vi "pulse destrbute_tester_1.vi"() -> ()   [LabVIEW 2021]
uses:
  Program Files/National Instruments/LabVIEW 2022/instr.lib/_niInstr/DSP/v1/Shared/Public/IQ Data.ctl
  Program Files/National Instruments/LabVIEW 2022/instr.lib/_niInstr/DSP/v1/Shared/niInstr DSP v1 Shared.lvlib
  pdw.ctl
panel:
  out "result 3":bool
  out "result 2":bool
  out "result":bool
  out "DDS free":bool[](array[boolean])=[FALSE, FALSE, FALSE, FALSE, FALSE, FALSE, FALSE, FALSE, FALSE, FALSE, FALSE, FALSE, FALSE, FALSE, FALSE, TRUE]
  in  "PDW":T1={"PW"=20, "frequency shift"=0.0, "amp"=0.9999923706054688, "mode type"=0, "mode file"=0, "mode depth"=0, "filter rate_pulse"=0, "filter rate bpsk"=0} {"frequency shift" format="%#_12f"}
  out "loop #":i32=421
  in  "stop":bool
  in  "new poulse":bool=TRUE
  in  "time good":bool=TRUE
  out "get new poulse":bool=TRUE
  out "output cluster":T2
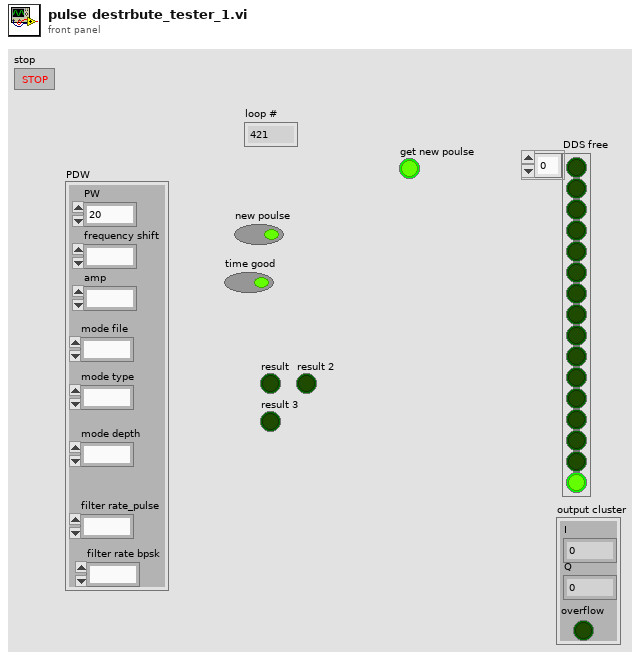
[diagram p1: front panel]
types:
  T1 = typedef "pdw.ctl" = cluster{"PW":u32, "frequency shift":fxp<+/-,48,0>, "amp":fxp<+/-,18,1>, "mode type":u8, "mode file":u8, "mode depth":u32, "filter rate_pulse":u16, "filter rate bpsk":u16}
  T2 = typedef "niInstr DSP v1 Shared.lvlib/IQ Data.ctl" = cluster{"I":fxp<+/-,18,1>, "Q":fxp<+/-,18,1>, "overflow":bool}
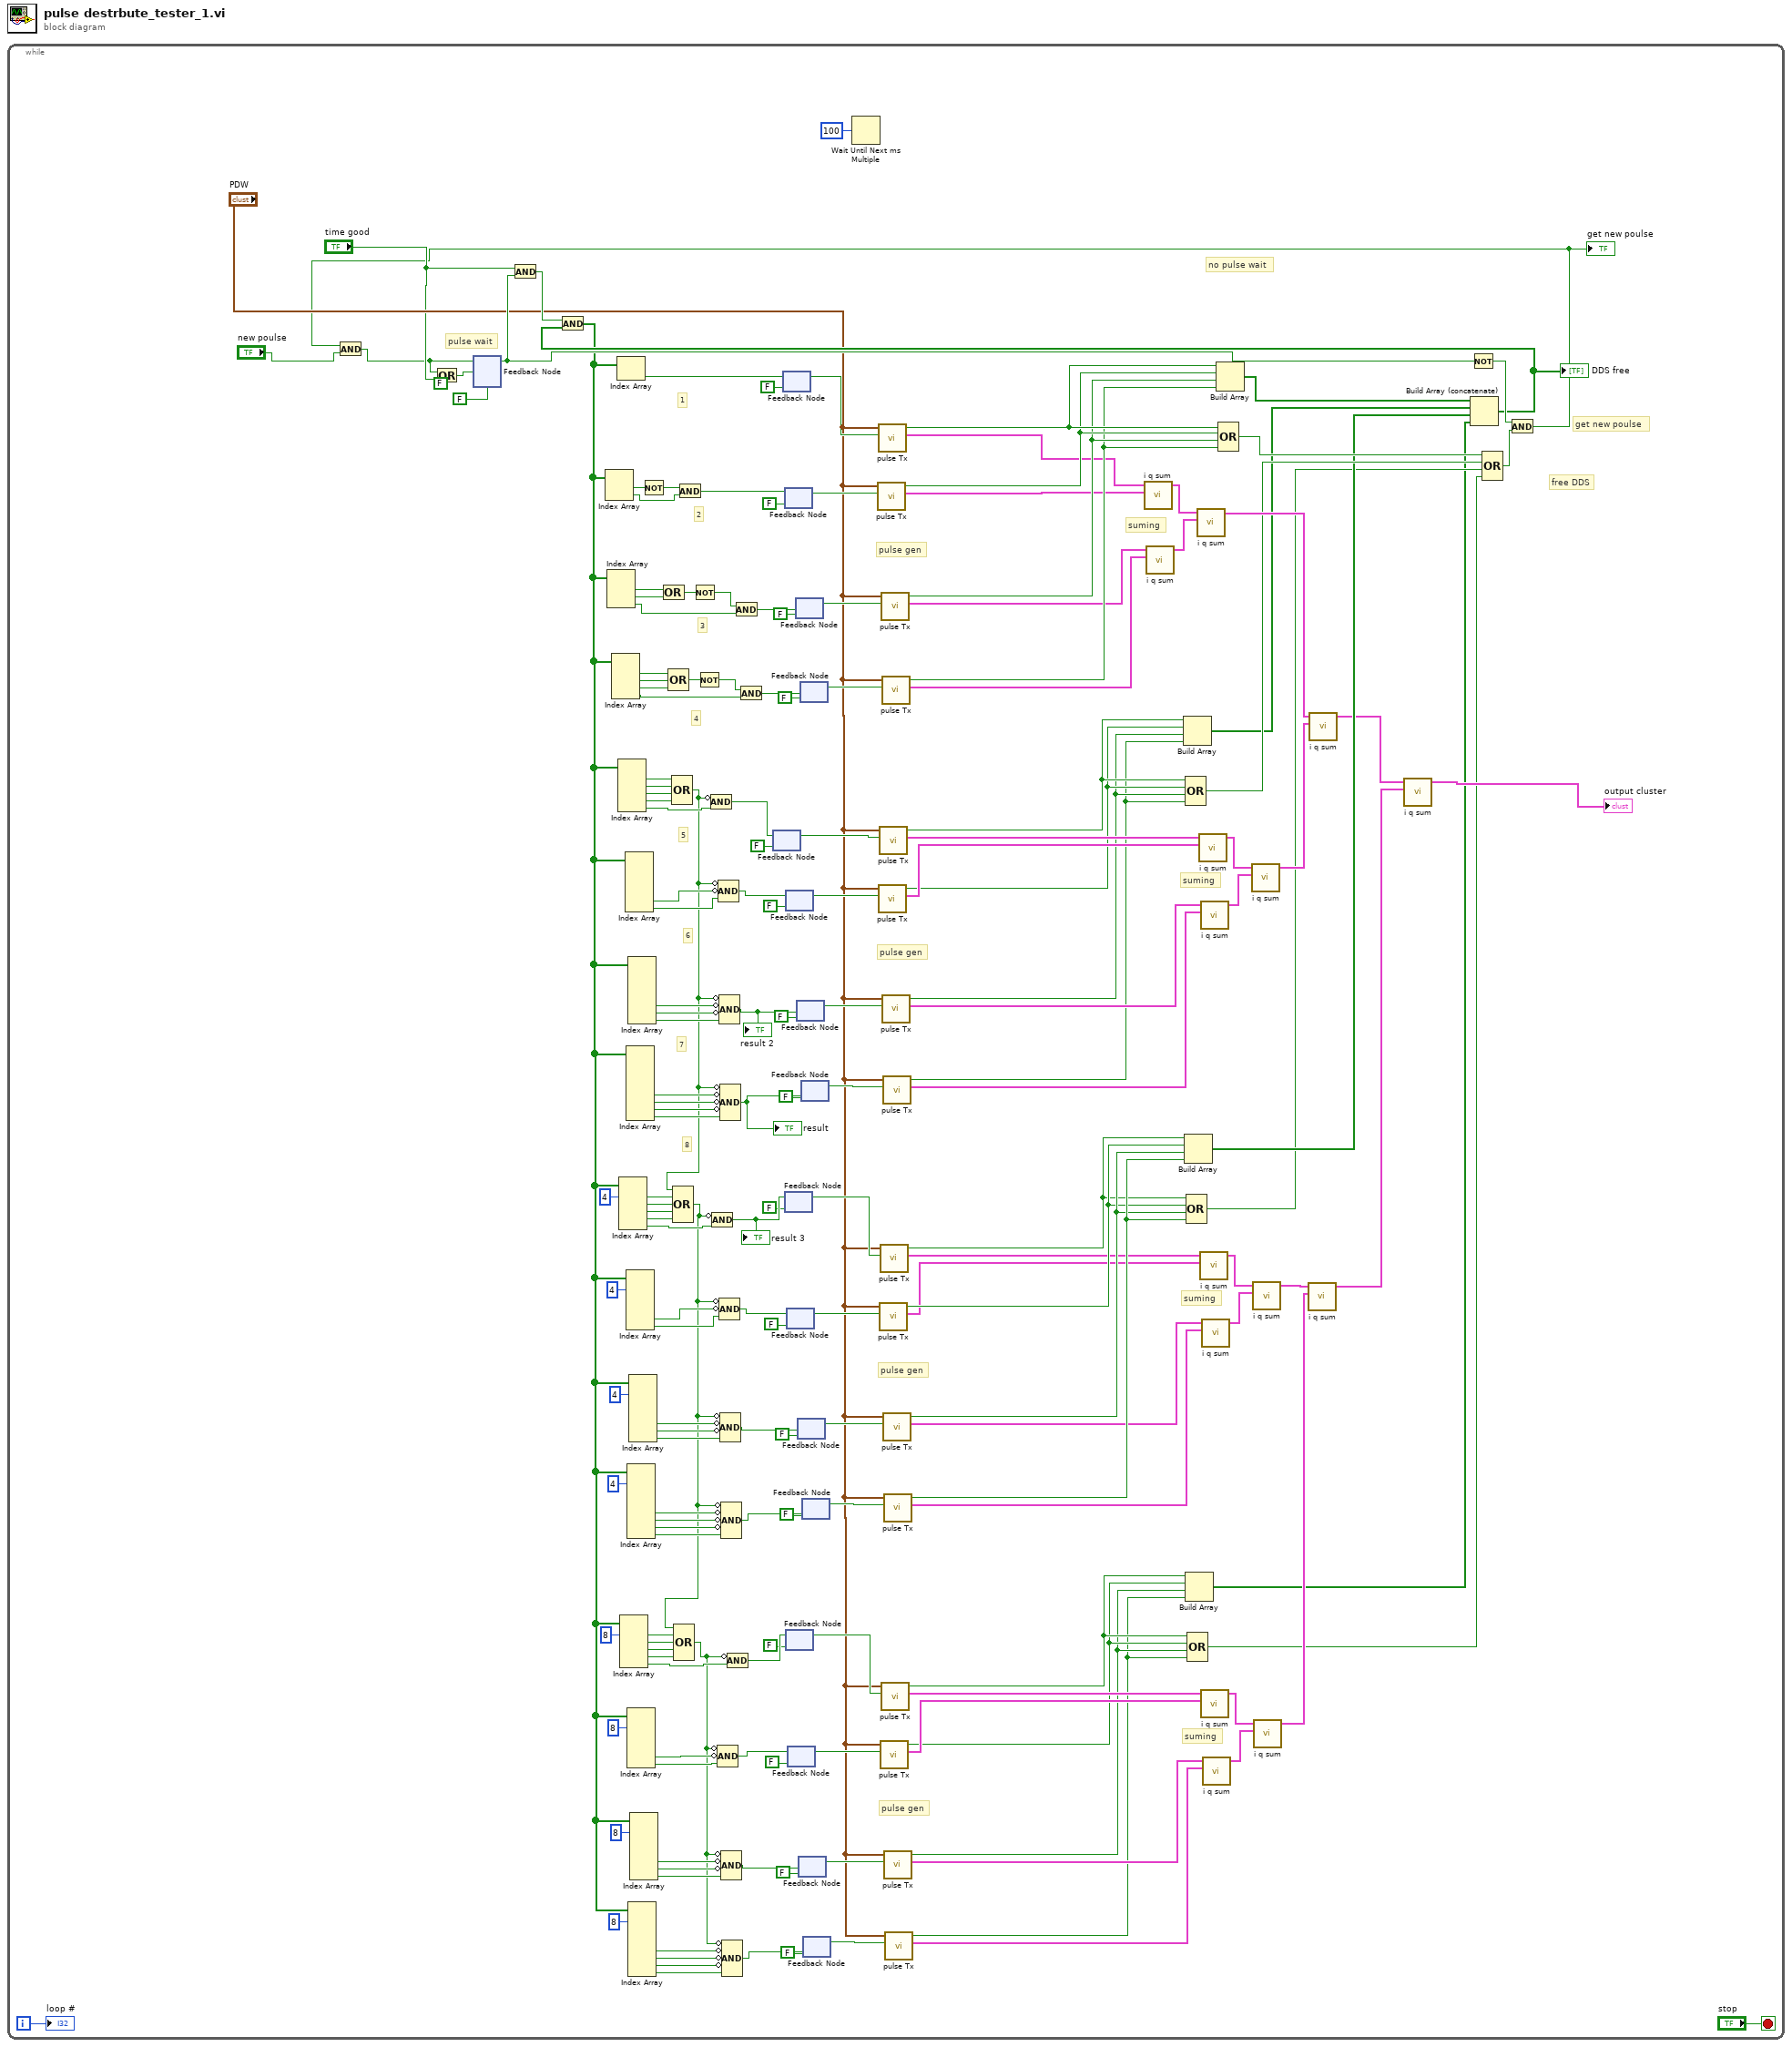
[diagram p0: block diagram]
diagram:
  n1 = while {
    i -> [w4]
    stop <- "stop" stop-if-true
    (unwired) FALSE ("Output Valid")
    # "8"
    # "7"
    # "6"
    # "5"
    # "4"
    # "3"
    # "2"
    # "1"
    # "suming"
    # "pulse gen"
    # "suming"
    # "pulse gen"
    # "suming"
    # "pulse gen"
    # "pulse wait"
    # "suming"
    # "pulse gen"
    # "get new poulse"
    # "no pulse wait"
    # "free DDS"
    n2 = feedback #1(FALSE ("Output Valid")) -> (w150:bool)
    n3 = And(x="time good", y=w150) -> (x .and. y?=w161:bool)
    n4 = feedback #2(FALSE) -> (w149:bool)
    n5 = feedback #3(FALSE) -> (w153:bool)
    n6 = feedback #4(FALSE) -> (w173:bool)
    n7 = feedback #5(FALSE) -> (w78:bool)
    n8 = feedback #6(FALSE) -> (w146:bool)
    n9 = feedback #7(FALSE) -> (w64:bool)
    n10 = feedback #8(FALSE) -> (w81:bool)
    n11 = feedback #9(FALSE) -> (w61:bool)
    n12 = feedback #10(FALSE) -> (w172:bool)
    n13 = feedback #11(FALSE) -> (w147:bool)
    n14 = feedback #12(FALSE) -> (w80:bool)
    n15 = feedback #13(FALSE) -> (w62:bool)
    n16 = feedback #14(FALSE) -> (w170:bool)
    n17 = feedback #15(FALSE) -> (w148:bool)
    n18 = feedback #16(FALSE) -> (w79:bool)
    n19 = feedback #17(FALSE) -> (w63:bool)
    n20 = Wait Until Next ms Multiple(millisecond multiple=u32 100) -> ()  [unwired: 1 out]
    n21 = call "pulse Tx.vi"("take it!"=w173, "Cluster"="PDW") -> ("data out"=w158:T2, "free dds"=w185:bool)  [unwired: 5 in, 3 out]
    n22 = call "pulse Tx.vi"("take it!"=w153, "Cluster"="PDW") -> ("data out"=w159:T2, "free dds"=w186:bool)  [unwired: 5 in, 3 out]
    n23 = call "pulse Tx.vi"("take it!"=w146, "Cluster"="PDW") -> ("data out"=w142:T2, "free dds"=w118:bool)  [unwired: 5 in, 3 out]
    n24 = call "pulse Tx.vi"("take it!"=w149, "Cluster"="PDW") -> ("data out"=w143:T2, "free dds"=w119:bool)  [unwired: 5 in, 3 out]
    n25 = call "pulse Tx.vi"("take it!"=w81, "Cluster"="PDW") -> ("data out"=w85:T2, "free dds"=w107:bool)  [unwired: 5 in, 3 out]
    n26 = call "pulse Tx.vi"("take it!"=w78, "Cluster"="PDW") -> ("data out"=w84:T2, "free dds"=w106:bool)  [unwired: 5 in, 3 out]
    n27 = call "pulse Tx.vi"("take it!"=w61, "Cluster"="PDW") -> ("data out"=w57:T2, "free dds"=w34:bool)  [unwired: 5 in, 3 out]
    n28 = call "pulse Tx.vi"("take it!"=w172, "Cluster"="PDW") -> ("data out"=w157:T2, "free dds"=w171:bool)  [unwired: 5 in, 3 out]
    n29 = call "pulse Tx.vi"("take it!"=w64, "Cluster"="PDW") -> ("data out"=w58:T2, "free dds"=w35:bool)  [unwired: 5 in, 3 out]
    n30 = call "pulse Tx.vi"("take it!"=w170, "Cluster"="PDW") -> ("data out"=w156:T2, "free dds"=w162:bool)  [unwired: 5 in, 3 out]
    n31 = call "pulse Tx.vi"("take it!"=w147, "Cluster"="PDW") -> ("data out"=w141:T2, "free dds"=w117:bool)  [unwired: 5 in, 3 out]
    n32 = call "pulse Tx.vi"("take it!"=w148, "Cluster"="PDW") -> ("data out"=w140:T2, "free dds"=w116:bool)  [unwired: 5 in, 3 out]
    n33 = call "pulse Tx.vi"("take it!"=w80, "Cluster"="PDW") -> ("data out"=w86:T2, "free dds"=w108:bool)  [unwired: 5 in, 3 out]
    n34 = call "pulse Tx.vi"("take it!"=w79, "Cluster"="PDW") -> ("data out"=w87:T2, "free dds"=w109:bool)  [unwired: 5 in, 3 out]
    n35 = call "pulse Tx.vi"("take it!"=w62, "Cluster"="PDW") -> ("data out"=w56:T2, "free dds"=w33:bool)  [unwired: 5 in, 3 out]
    n36 = call "pulse Tx.vi"("take it!"=w63, "Cluster"="PDW") -> ("data out"=w55:T2, "free dds"=w32:bool)  [unwired: 5 in, 3 out]
    n37 = call "i q sum.vi"(10:"data in"=w158, 11:"data in"=w159) -> ("output cluster"=w155:T2)  [unwired: 8 in, 1 out]
    n38 = call "i q sum.vi"(10:"data in"=w156, 11:"data in"=w157) -> ("output cluster"=w154:T2)  [unwired: 8 in, 1 out]
    n39 = Build Array(w119, w118, w117, w116) -> (w111:bool[])
    n40 = Build Array(w106, w107, w108, w109) -> (w72:bool[])
    n41 = Compound Arithmetic op=OR(w119, w118, w117, w116) -> (w114:bool)
    n42 = Build Array(w35, w34, w33, w32) -> (w27:bool[])
    n43 = Compound Arithmetic op=OR(w106, w107, w108, w109) -> (w71:bool)
    n44 = Compound Arithmetic op=OR(w35, w34, w33, w32) -> (w26:bool)
    n45 = call "i q sum.vi"(10:"data in"=w154, 11:"data in"=w155) -> ("output cluster"=w121:T2)  [unwired: 8 in, 1 out]
    n46 = call "i q sum.vi"(10:"data in"=w142, 11:"data in"=w143) -> ("output cluster"=w144:T2)  [unwired: 8 in, 1 out]
    n47 = call "i q sum.vi"(10:"data in"=w85, 11:"data in"=w84) -> ("output cluster"=w83:T2)  [unwired: 8 in, 1 out]
    n48 = call "i q sum.vi"(10:"data in"=w140, 11:"data in"=w141) -> ("output cluster"=w145:T2)  [unwired: 8 in, 1 out]
    n49 = call "i q sum.vi"(10:"data in"=w57, 11:"data in"=w58) -> ("output cluster"=w59:T2)  [unwired: 8 in, 1 out]
    n50 = call "i q sum.vi"(10:"data in"=w87, 11:"data in"=w86) -> ("output cluster"=w82:T2)  [unwired: 8 in, 1 out]
    n51 = call "i q sum.vi"(10:"data in"=w55, 11:"data in"=w56) -> ("output cluster"=w60:T2)  [unwired: 8 in, 1 out]
    n52 = Build Array(w186, w185, w171, w162) -> (w112:bool[])
    n53 = Compound Arithmetic op=OR(w186, w185, w171, w162) -> (w115:bool)
    n54 = call "i q sum.vi"(10:"data in"=w145, 11:"data in"=w144) -> ("output cluster"=w120:T2)  [unwired: 8 in, 1 out]
    n55 = call "i q sum.vi"(10:"data in"=w82, 11:"data in"=w83) -> ("output cluster"=w30:T2)  [unwired: 8 in, 1 out]
    n56 = call "i q sum.vi"(10:"data in"=w60, 11:"data in"=w59) -> ("output cluster"=w29:T2)  [unwired: 8 in, 1 out]
    n57 = call "i q sum.vi"(10:"data in"=w29, 11:"data in"=w30) -> ("output cluster"=w28:T2)  [unwired: 8 in, 1 out]
    n58 = call "i q sum.vi"(10:"data in"=w120, 11:"data in"=w121) -> ("output cluster"=w70:T2)  [unwired: 8 in, 1 out]
    n59 = call "i q sum.vi"(10:"data in"=w28, 11:"data in"=w70) -> ("output cluster"=→"output cluster":T2)  [unwired: 8 in, 1 out]
    n60 = Not(x=w150) -> (.not. x?=w160:bool)
    n61 = Build Array (concatenate)(w112, w111, w72, w27) -> (w110:bool[])
    "DDS free" <- w110
    n62 = And(x=w161, y=w110) -> (x .and. y?=w31:bool[])
    n63 = Index Array(array=w31) -> (element #1=w183:bool, element #2=w181:bool)  [unwired: 2 in]
    n64 = Index Array(array=w31) -> (element #1=w175:bool, element #2=w176:bool, element #3=w177:bool)  [unwired: 3 in]
    n65 = Index Array(array=w31) -> (element #1=w168:bool, element #2=w167:bool, element #3=w163:bool, element #4=w164:bool)  [unwired: 4 in]
    n66 = Index Array(array=w31) -> (element=w184:bool)  [unwired: 1 in]
    n67 = Index Array(array=w31) -> (element #1=w139:bool, element #2=w138:bool, element #3=w137:bool, element #4=w136:bool, element #5=w135:bool)  [unwired: 5 in]
    n68 = Index Array(array=w31, index #1=4 ("index")) -> (element #1=w88:bool, element #2=w89:bool, element #3=w90:bool, element #4=w91:bool, element #5=w92:bool)  [unwired: 4 in]
    n69 = Index Array(array=w31, index #1=8 ("index")) -> (element #1=w54:bool, element #2=w53:bool, element #3=w52:bool, element #4=w51:bool, element #5=w50:bool)  [unwired: 4 in]
    n70 = Index Array(array=w31) -> (element #5=w131:bool, element #6=w133:bool)  [unwired: 6 in, 4 out]
    n71 = Index Array(array=w31) -> (element #5=w123:bool, element #6=w124:bool, element #7=w125:bool, element #8=w126:bool)  [unwired: 8 in, 4 out]
    n72 = Index Array(array=w31, index #1=4 ("index")) -> (element #5=w96:bool, element #6=w94:bool)  [unwired: 5 in, 4 out]
    n73 = Index Array(array=w31, index #1=4 ("index")) -> (element #5=w104:bool, element #6=w103:bool, element #7=w102:bool, element #8=w101:bool)  [unwired: 7 in, 4 out]
    n74 = Index Array(array=w31, index #1=8 ("index")) -> (element #5=w46:bool, element #6=w48:bool)  [unwired: 5 in, 4 out]
    n75 = Index Array(array=w31) -> (element #5=w127:bool, element #6=w128:bool, element #7=w129:bool)  [unwired: 7 in, 4 out]
    n76 = Index Array(array=w31, index #1=8 ("index")) -> (element #5=w38:bool, element #6=w39:bool, element #7=w40:bool, element #8=w41:bool)  [unwired: 7 in, 4 out]
    n77 = Index Array(array=w31, index #1=4 ("index")) -> (element #5=w100:bool, element #6=w99:bool, element #7=w98:bool)  [unwired: 6 in, 4 out]
    n78 = Index Array(array=w31, index #1=8 ("index")) -> (element #5=w42:bool, element #6=w43:bool, element #7=w44:bool)  [unwired: 6 in, 4 out]
    n79 = Not(x=w183) -> (.not. x?=w182:bool)
    n80 = Compound Arithmetic op=OR(w175, w176) -> (w174:bool)
    n81 = Compound Arithmetic op=OR(w168, w167, w163) -> (w169:bool)
    n82 = Compound Arithmetic op=OR(w139, w138, w137, w136) -> (w76:bool)
    n83 = Compound Arithmetic op=OR(w76, w88, w89, w90, w91) -> (w25:bool)
    n84 = Compound Arithmetic op=OR(w25, w54, w53, w52, w51) -> (w37:bool)
    n85 = And(x=w182, y=w181) -> (x .and. y?=w180:bool)
    n86 = Not(x=w174) -> (.not. x?=w178:bool)
    n87 = Not(x=w169) -> (.not. x?=w166:bool)
    n88 = Compound Arithmetic op=AND(invert w76, w135) -> (w134:bool)
    n89 = Compound Arithmetic op=AND(invert w25, w92) -> (w93:bool)
    "result 3" <- w93
    n90 = Compound Arithmetic op=AND(invert w37, invert w46, w48) -> (w47:bool)
    n91 = Compound Arithmetic op=AND(invert w76, invert w131, w133) -> (w132:bool)
    n92 = Compound Arithmetic op=AND(invert w76, invert w127, invert w128, w129) -> (w130:bool)
    "result 2" <- w130
    n93 = Compound Arithmetic op=AND(invert w25, invert w96, w94) -> (w95:bool)
    n94 = Compound Arithmetic op=AND(invert w76, invert w123, invert w124, invert w125, w126) -> (w122:bool)
    "result" <- w122
    n95 = Compound Arithmetic op=AND(invert w25, invert w100, invert w99, w98) -> (w97:bool)
    n96 = Compound Arithmetic op=AND(invert w25, invert w104, invert w103, invert w102, w101) -> (w105:bool)
    n97 = Compound Arithmetic op=AND(invert w37, invert w42, invert w43, w44) -> (w45:bool)
    n98 = Compound Arithmetic op=AND(invert w37, invert w38, invert w39, invert w40, w41) -> (w36:bool)
    n99 = Compound Arithmetic op=AND(invert w37, w50) -> (w49:bool)
    n100 = And(x=w178, y=w177) -> (x .and. y?=w179:bool)
    n101 = And(x=w166, y=w164) -> (x .and. y?=w165:bool)
    n102 = feedback-in #2(w134) -> ()
    n103 = feedback-in #3(w184) -> ()
    n104 = feedback-in #4(w180) -> ()
    n105 = feedback-in #5(w93) -> ()
    n106 = feedback-in #6(w132) -> ()
    n107 = feedback-in #7(w49) -> ()
    n108 = feedback-in #8(w95) -> ()
    n109 = feedback-in #9(w47) -> ()
    n110 = feedback-in #10(w179) -> ()
    n111 = feedback-in #11(w130) -> ()
    n112 = feedback-in #12(w97) -> ()
    n113 = feedback-in #13(w45) -> ()
    n114 = feedback-in #14(w165) -> ()
    n115 = feedback-in #15(w122) -> ()
    n116 = feedback-in #16(w105) -> ()
    n117 = feedback-in #17(w36) -> ()
    n118 = Compound Arithmetic op=OR(w115, w114, w71, w26) -> (w113:bool)
    n119 = And(x=w160, y=w113) -> (x .and. y?=w3:bool)
    "get new poulse" <- w3
    n120 = And(x=w3, y="new poulse") -> (x .and. y?=w1:bool)
    n121 = Or(x=w1, y="time good") -> (x .or. y?=w151:bool)
    n122 = feedback-in #1(w1, w151) -> ()
    "loop #" <- w4
  }
